vi "createStatementToDBInUpdateVI.vi"(7 "DataReadingInTableBeforeToUpdate":string[][](array[string]), 8 "Nombre Tabla":string, 9 "ColumnName":string[](array[string]), 10 "RawIndexToModify":i32[](array[numeric]), 11 "ItemNames":string[][](array[string])) -> (0 "DataToModify5":T2, 1 "TableNameToModify":string, 2 "DataToModify3":T1, 3 "statementSQL":string, 5 "NumberOfFields":i32)   [LabVIEW 2014]
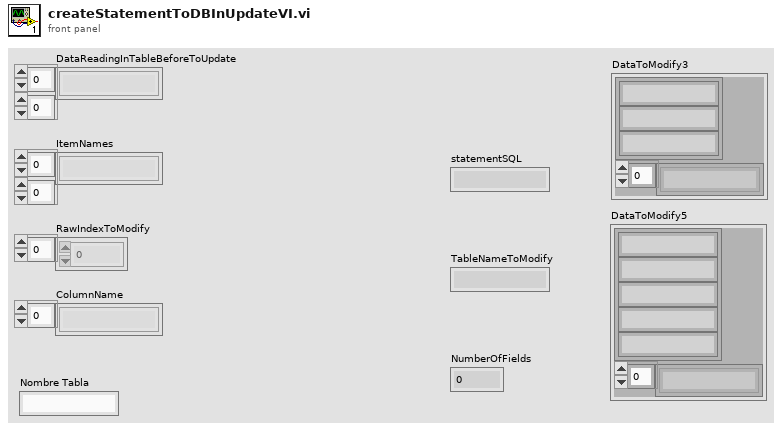
[diagram p1: front panel]
types:
  T1 = cluster{cluster{string, string, string}, string[]}
  T2 = cluster{cluster{string, string, string, string, string}, string[]}
  T3 = cluster{string, string, "StringTimeMySQLFormat":string}
  T4 = cluster{cluster{string, string, "StringTimeMySQLFormat":string}, string[]}
  T5 = cluster{string, string, string, string, "StringTimeMySQLFormat":string}
  T6 = cluster{cluster{string, string, string, string, "StringTimeMySQLFormat":string}, string[]}
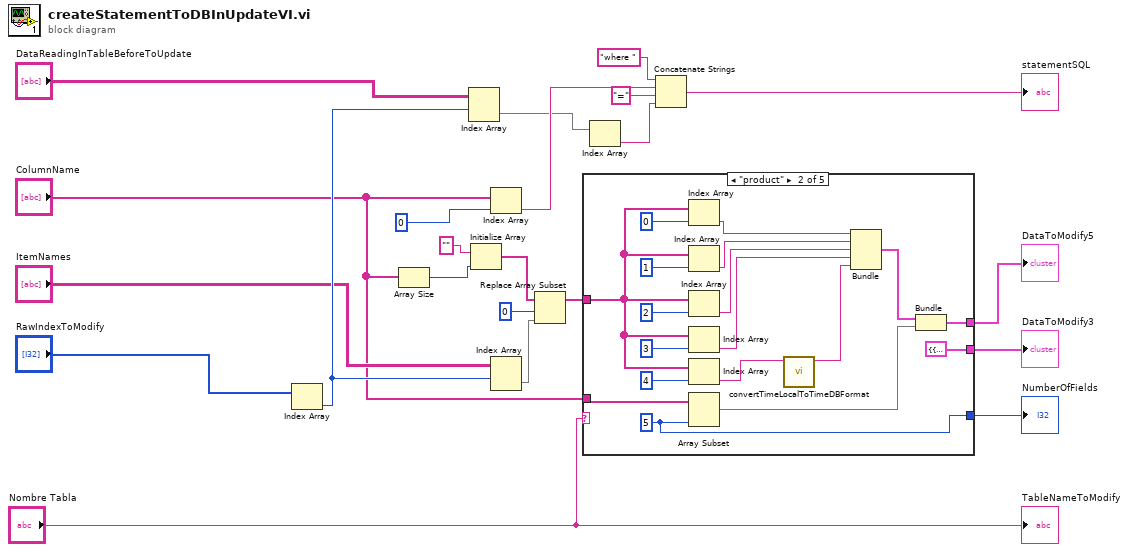
[diagram p0: block diagram]
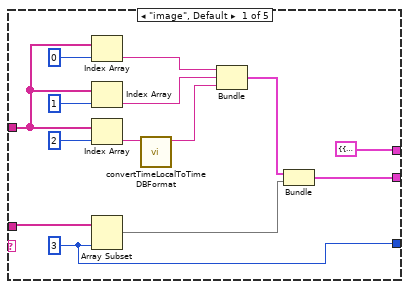
[diagram p2: hidden frame]
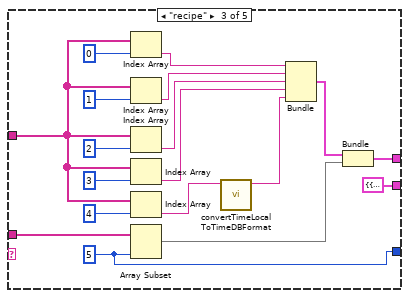
[diagram p3: hidden frame]
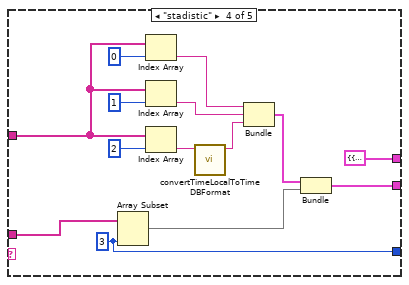
[diagram p4: hidden frame]
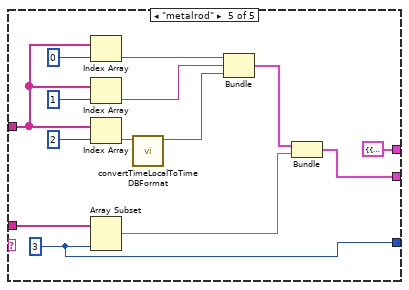
[diagram p5: hidden frame]
diagram:
  n1 = Index Array(array="RawIndexToModify") -> (element=w16:i32)  [unwired: 1 in]
  n2 = Array Size(array="ColumnName") -> (size(s)=w13:i32)
  n3 = Index Array(array="DataReadingInTableBeforeToUpdate", index (row)=w16) -> (element=w17:string[])  [unwired: 1 in]
  n4 = Initialize Array("", w13) -> (w12:string[])
  n5 = Index Array(array="ColumnName", index=0) -> (element=w19:string)
  n6 = Index Array(array="ItemNames", index (row)=w16) -> (element=w14:string[])  [unwired: 1 in]
  n7 = Replace Array Subset(array=w12, new element=w14, index=0) -> (w7:string[])
  n8 = case shown="\"product\"" "Nombre Tabla" {
    tunnel: w7 -> [w31 w46 w61 w83 w100]
    tunnel: "ColumnName" -> [w30 w44 w60 w82 w94]
    tunnel: [T2 {{"", "", "", "", ""}, []} w41 w59 T2 {{"", "", "", "", ""}, []} T2 {{"", "", "", "", ""}, []}] -> w4
    tunnel: [w27 T1 {{"", "", ""}, []} T1 {{"", "", ""}, []} w77 w91] -> w3
    tunnel: [w25 w39 w57 w75 w89] -> w2
    frame "image", Default {
      w25 = 3 ("length")
      n9 = Index Array(array=w31, index=0) -> (element=w34:string)
      n10 = Index Array(array=w31, index=1) -> (element=w33:string)
      n11 = Index Array(array=w31, index=2) -> (element=w24:string)
      n12 = Array Subset(array=w30, length=w25) -> (w28:string[])  [unwired: 1 in]
      n13 = call "convertTimeLocalToTimeDBFormat.vi"("StringTimeLocalFormat"=w24) -> ("StringTimeMySQLFormat"=w23:string)  [unwired: 10 in]
      n14 = Bundle(w34, w33, "StringTimeMySQLFormat"=w23) -> (w29:T3)  [unwired: 1 in]
      n15 = Bundle(w29, w28) -> (w27:T4)  [unwired: 1 in]
    }
    frame "product" {
      w39 = 5 ("length")
      n16 = Index Array(array=w46, index=0) -> (element=w52:string)
      n17 = Index Array(array=w46, index=1) -> (element=w51:string)
      n18 = Index Array(array=w46, index=2) -> (element=w49:string)
      n19 = Index Array(array=w46, index=3) -> (element=w45:string)
      n20 = Index Array(array=w46, index=4) -> (element=w38:string)
      n21 = Array Subset(array=w44, length=w39) -> (w42:string[])  [unwired: 1 in]
      n22 = call "convertTimeLocalToTimeDBFormat.vi"("StringTimeLocalFormat"=w38) -> ("StringTimeMySQLFormat"=w37:string)  [unwired: 10 in]
      n23 = Bundle(w52, w51, w49, w45, "StringTimeMySQLFormat"=w37) -> (w43:T5)  [unwired: 1 in]
      n24 = Bundle(w43, w42) -> (w41:T6)  [unwired: 1 in]
    }
    frame "recipe" {
      w57 = 5 ("length")
      n25 = Index Array(array=w61, index=0) -> (element=w70:string)
      n26 = Index Array(array=w61, index=1) -> (element=w69:string)
      n27 = Index Array(array=w61, index=2) -> (element=w67:string)
      n28 = Index Array(array=w61, index=3) -> (element=w64:string)
      n29 = Index Array(array=w61, index=4) -> (element=w56:string)
      n30 = Array Subset(array=w60, length=w57) -> (w62:string[])  [unwired: 1 in]
      n31 = call "convertTimeLocalToTimeDBFormat.vi"("StringTimeLocalFormat"=w56) -> ("StringTimeMySQLFormat"=w55:string)  [unwired: 10 in]
      n32 = Bundle(w70, w69, w67, w64, "StringTimeMySQLFormat"=w55) -> (w63:T5)  [unwired: 1 in]
      n33 = Bundle(w63, w62) -> (w59:T6)  [unwired: 1 in]
    }
    frame "stadistic" {
      w75 = 3 ("length")
      n34 = Array Subset(array=w82, length=w75) -> (w78:string[])  [unwired: 1 in]
      n35 = Index Array(array=w83, index=0) -> (element=w80:string)
      n36 = Index Array(array=w83, index=1) -> (element=w79:string)
      n37 = Index Array(array=w83, index=2) -> (element=w74:string)
      n38 = call "convertTimeLocalToTimeDBFormat.vi"("StringTimeLocalFormat"=w74) -> ("StringTimeMySQLFormat"=w73:string)  [unwired: 10 in]
      n39 = Bundle(w80, w79, "StringTimeMySQLFormat"=w73) -> (w81:T3)  [unwired: 1 in]
      n40 = Bundle(w81, w78) -> (w77:T4)  [unwired: 1 in]
    }
    frame "metalrod" {
      w89 = 3 ("length")
      n41 = Index Array(array=w100, index=0) -> (element=w96:string)
      n42 = Index Array(array=w100, index=1) -> (element=w95:string)
      n43 = Index Array(array=w100, index=2) -> (element=w88:string)
      n44 = Array Subset(array=w94, length=w89) -> (w92:string[])  [unwired: 1 in]
      n45 = call "convertTimeLocalToTimeDBFormat.vi"("StringTimeLocalFormat"=w88) -> ("StringTimeMySQLFormat"=w87:string)  [unwired: 10 in]
      n46 = Bundle(w96, w95, "StringTimeMySQLFormat"=w87) -> (w93:T3)  [unwired: 1 in]
      n47 = Bundle(w93, w92) -> (w91:T4)  [unwired: 1 in]
    }
  }
  "DataToModify5" <- w4
  "DataToModify3" <- w3
  "NumberOfFields" <- w2
  n48 = Index Array(array=w17) -> (element=w21:string)  [unwired: 1 in]
  n49 = Concatenate Strings("where " ("condition"), w19, "=" ("string"), w21) -> (→"statementSQL":string)
  "TableNameToModify" <- "Nombre Tabla"
